vi "Load Transactions.vi"(8 "error in (no error)":errorcluster, 11 "Budgetizer in":refnum<class "Budgetizer.lvclass">) -> (0 "error out":errorcluster, 3 "Budgetizer out":refnum<class "Budgetizer.lvclass">)   [LabVIEW 2018, in "Budgetizer.lvclass"]
uses:
  Budgetizer.lvclass
  Budgetizer.lvclass/Budgetizer.ctl
  database/Database.lvclass
  Statement/Statement.lvclass
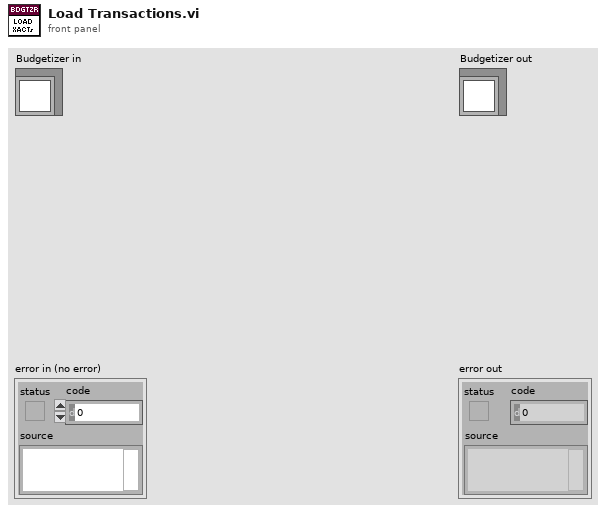
[diagram p1: front panel]
types:
  T1 = typedef "LVDateTimeRec.ctl" = cluster{"fractional second":dbl, "second":i32, "minute":i32, "hour":i32, "day of month":i32, "month":i32, "year":i32, "day of week":i32, "day of year":i32, "DST":i32}
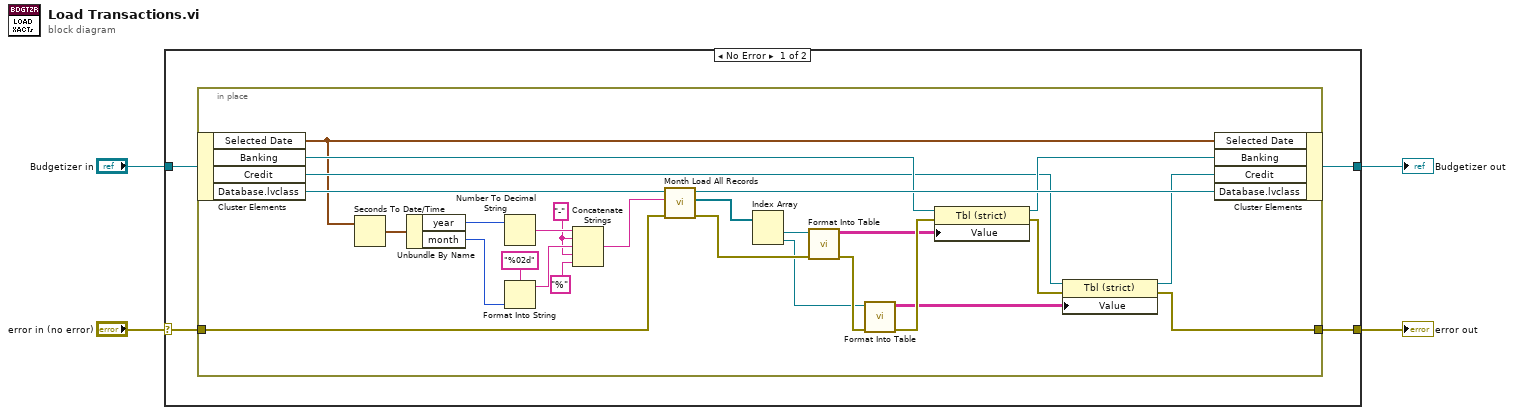
[diagram p0: block diagram]
diagram:
  n1 = case shown="No Error" "error in (no error)" {
    selector: "error in (no error)" -> [w8 w37]
    tunnel: [w7 w37] -> w3
    tunnel: [w5 w36] -> w1
    tunnel: "Budgetizer in" -> [w6 w36]
    frame No Error {
      n2 = in-place {
        in-place-border: w8 -> [w31]
        in-place-border: [w20] -> w7
        w14 = "-" ("string")
        n3 = in-place-cluster #1(w6) -> ("Selected Date"=w18:timestamp, "Banking"=w27:refnum<vi>, "Credit"=w22:refnum<vi>, "Database.lvclass"=w30:refnum<class "Database.lvclass">)
        n4 = Seconds To Date/Time(time stamp (now)=w18) -> (date time rec=w12:T1)  [unwired: 1 in]
        n5 = Unbundle By Name(w12) -> ("year"=w11:i32, "month"=w10:i32)
        n6 = Number To Decimal String(number=w11) -> (decimal integer string=w17:string)  [unwired: 1 in]
        n7 = Format Into String(format string="%02d" ("string"), w10) -> (resulting string=w15:string)  [unwired: 2 in, 1 out]
        n8 = Concatenate Strings(w17, w14, w15, w14, "%" ("string")) -> (w9:string)
        n9 = call "Month Load All Records.vi"("error in (no error)"=w31, "SQL Date"=w9, "Database in"=w30) -> ("error out"=w34:errorcluster, "Statements"=w19:refnum<class "Statement.lvclass">[], "Database out"=w29:refnum<class "Database.lvclass">)  [unwired: 6 in]
        n10 = Index Array(array=w19) -> (element #1=w35:refnum<class "Statement.lvclass">, element #2=w32:refnum<class "Statement.lvclass">)  [unwired: 2 in]
        n11 = call "Format Into Table.vi"("error in (no error)"=w34, "Statement in"=w35) -> ("error out"=w33:errorcluster, "Table Row"=w26:string[][])  [unwired: 8 in]
        n12 = call "Format Into Table.vi"("error in (no error)"=w33, "Statement in"=w32) -> ("error out"=w28:errorcluster, "Table Row"=w24:string[][])  [unwired: 8 in]
        n13 = property class="Tbl (strict)"(reference=w27, error in=w28, "Value"=w26) -> (reference out=w25:refnum<vi>, error out=w23:errorcluster)
        n14 = property class="Tbl (strict)"(reference=w22, error in=w23, "Value"=w24) -> (reference out=w21:refnum<vi>, error out=w20:errorcluster)
        n15 = in-place-cluster #1("Selected Date"=w18, "Banking"=w25, "Credit"=w21, "Database.lvclass"=w29) -> (w5:refnum<class "Budgetizer.lvclass">)
      }
    }
    frame Error {
    }
  }
  "error out" <- w3
  "Budgetizer out" <- w1
